vi "Cable Length.vi"(6 "Encoder Initialize":bool, 9 "Compensation in":dbl[](array[numeric]), 10 "Encoder Position":dbl[](array[numeric]), 11 "Initial Cable Length":dbl[](array[numeric])) -> (2 "Cable Length out":dbl[](array[numeric]), 3 "Compensation out":dbl[](array[numeric]))   [LabVIEW 2021]
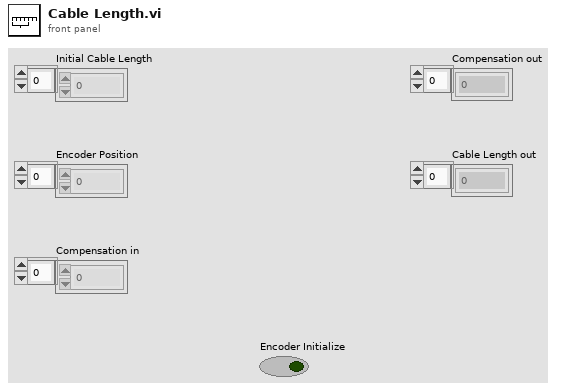
[diagram p1: front panel]
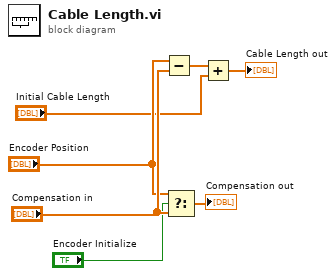
[diagram p0: block diagram]
diagram:
  n1 = Subtract(x="Encoder Position", y="Compensation in") -> (x-y=w2:dbl[])
  n2 = Select(t="Encoder Position", s="Encoder Initialize", f="Compensation in") -> (s? t:f=→"Compensation out":dbl[])
  n3 = Add(x=w2, y="Initial Cable Length") -> (x+y=→"Cable Length out":dbl[])
